vi "DIO_PWM_Encoder_I2C.vi"(0 "DIO.1:0.OUT":fxp<+,2,2> format="%.0b", 1 "DIO.1:0.DIR":fxp<+,2,2> format="%.0b", 3 "PWM.GROUP IN":T3 {"PWM.1.CNFG" format="%08b"; "PWM.0.CNFG" format="%08b"}, 4 "Encoder.GROUP IN":T4 {"ENC.STAT" format="%08b"}, 5 "I2C.GROUP IN":T1={"I2C.GO"=FALSE, "I2C.CNFG"=1, "I2C.DATO"=0, "I2C.DATI"=0, "I2C.ADDR"=0, "I2C.CNTR"=213, "I2C.CNTL"=0, "I2C.STAT"=0} {"I2C.STAT" format="%08b"; "I2C.CNTL" format="%08b"; "I2C.ADDR" format="%08b"; "I2C.CNFG" format="%08b"}, 6 "DIO0/PWM0/ENC.A/I2C.SCL Refnum":refnum<k21>, 7 "DIO.1:0.Selector":fxp<+,4,4> format="%.0b", 8 "DIO1/PWM1/ENC.B/I2C.SDA Refnum":refnum<k21>) -> (14 "IN 1:0":fxp<+,2,2> format="%02b", 17 "PWM.GROUP OUT":T3 {"PWM.1.CNFG" format="%08b"; "PWM.0.CNFG" format="%08b"}, 18 "Encoder.GROUP OUT":T4 {"ENC.STAT" format="%08b"}, 19 "I2C.GROUP OUT":T1={"I2C.GO"=FALSE, "I2C.CNFG"=1, "I2C.DATO"=0, "I2C.DATI"=0, "I2C.ADDR"=0, "I2C.CNTR"=213, "I2C.CNTL"=0, "I2C.STAT"=0} {"I2C.STAT" format="%08b"; "I2C.CNTL" format="%08b"; "I2C.ADDR" format="%08b"; "I2C.CNFG" format="%08b"})   [LabVIEW 2019]
uses:
  Utilities/PWM Configuration Group.ctl
  Utilities/Encoder Configuration Group.ctl
  Utilities/I2C Configuration Group.ctl
  Utilities/Start Boolean.ctl
  <vilib>/rvi/eio/common/nirviEmuTemplateMethod_errors.vi
  <vilib>/eio/EIONode/EIONode.xnode
panel:
  # "This VI switches between the DIO functionality and the PWM/Encoder/I2C functionality for the specified FPGA I/O channels. Each bit has a selector which contains two-bits booleans.\n- If SELECT 0 is 00, DIO enabled.\n- If SELECT 0 is 01, PWM enabled.\n- If SELECT 0 is 10, Encoder enabled.\n- If SELECT 0 is 11, I2C enabled."
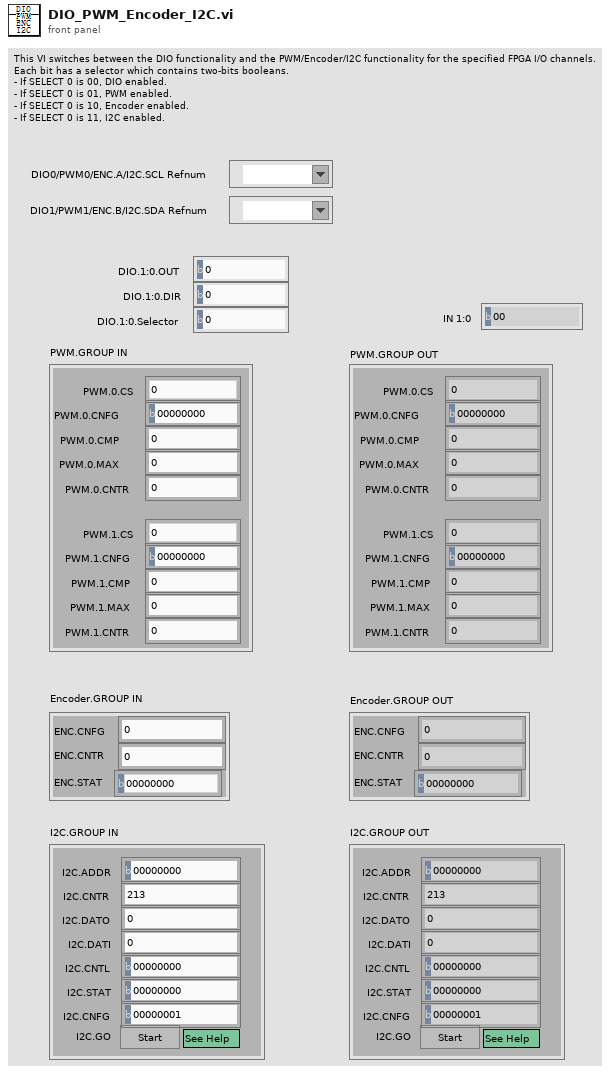
[diagram p1: front panel]
types:
  T1 = typedef "I2C Configuration Group.ctl" = cluster{"I2C.GO":T2, "I2C.CNFG":u8, "I2C.DATO":u8, "I2C.DATI":u8, "I2C.ADDR":u8, "I2C.CNTR":u8, "I2C.CNTL":u8, "I2C.STAT":u8}
  T2 = typedef "Start Boolean.ctl" = bool
  T3 = typedef "PWM Configuration Group.ctl" = cluster{"PWM.0.CS":u8, "PWM.0.CNFG":u8, "PWM.0.CMP":u16, "PWM.0.MAX":u16, "PWM.0.CNTR":u16, "PWM.1.CS":u8, "PWM.1.CNFG":u8, "PWM.1.CMP":u16, "PWM.1.MAX":u16, "PWM.1.CNTR":u16}
  T4 = typedef "Encoder Configuration Group.ctl" = cluster{"ENC.CNFG":u8, "ENC.CNTR":u32, "ENC.STAT":u8}
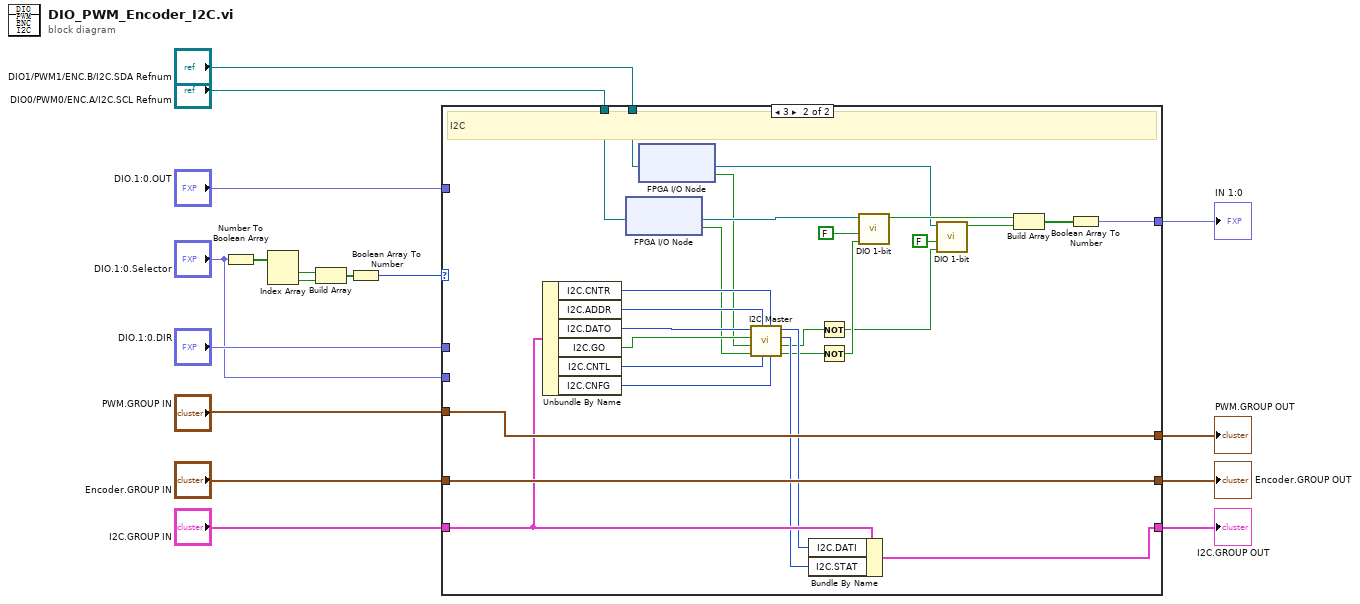
[diagram p0: block diagram]
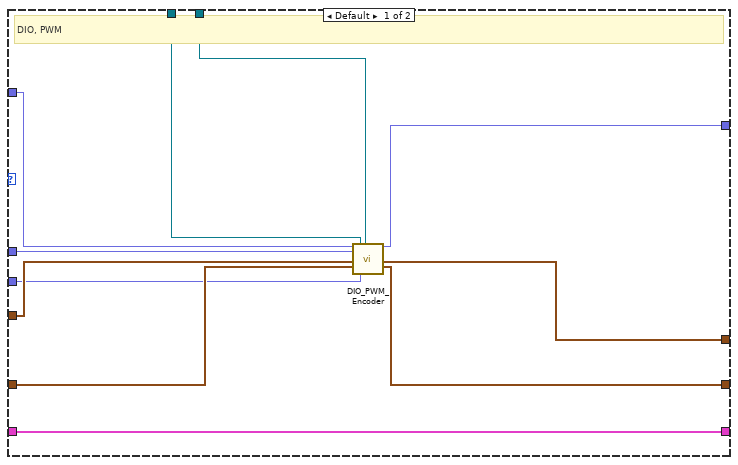
[diagram p2: hidden frame]
diagram:
  n1 = Number To Boolean Array(number="DIO.1:0.Selector") -> (Boolean array=w17:bool[])
  n2 = Index Array(array=w17) -> (element #1=w6:bool, element #2=w16:bool)  [unwired: 2 in]
  n3 = Build Array(w6, w16) -> (w15:bool[])
  n4 = Boolean Array To Number(Boolean array=w15) -> (number=w11:u8)
  n5 = case shown="3" w11 {
    tunnel: "PWM.GROUP IN" -> [w25 w55]
    tunnel: "Encoder.GROUP IN" -> [w24 w56]
    tunnel: [w22 w55] -> w12
    tunnel: [w21 w56] -> w7
    tunnel: [w23 w37] -> w10
    tunnel: "DIO0/PWM0/ENC.A/I2C.SCL Refnum" -> [w28 w36]
    tunnel: "DIO1/PWM1/ENC.B/I2C.SDA Refnum" -> [w27 w34]
    tunnel: "I2C.GROUP IN" -> [w19 w48]
    tunnel: [w19 w47] -> w4
    tunnel: "DIO.1:0.DIR" -> [w26 _]
    tunnel: "DIO.1:0.Selector" -> [w20 _]
    tunnel: "DIO.1:0.OUT" -> [w18 _]
    frame Default {
      # "DIO, PWM"
      n6 = call "DIO_PWM_Encoder.vi"("DIO.1:0.OUT"=w18, "DIO.1:0.DIR"=w26, "PWM.GROUP IN"=w25, "Encoder.GROUP IN"=w24, "DIO0/PWM0/ENC.A Refnum"=w28, "DIO.1:0.Selector"=w20, "DIO1/PWM1/ENC.B Refnum"=w27) -> ("IN 1:0"=w23:fxp<+,2,2>, "PWM.GROUP OUT"=w22:T3, "Encoder.GROUP OUT"=w21:T4)  [unwired: 10 in]
    }
    frame 3 {
      # "I2C"
      n7 = Unbundle By Name(w48) -> ("I2C.CNTR"=w54:u8, "I2C.ADDR"=w53:u8, "I2C.DATO"=w52:u8, "I2C.GO"=w51:T2, "I2C.CNTL"=w50:u8, "I2C.CNFG"=w49:u8)
      n8 = xnode "FPGA I/O Node"("FPGA I/O输入"=w36) -> ("I/O项"=w32:bool, "FPGA I/O输出"=w35:refnum<k21>)
      n9 = xnode "FPGA I/O Node"("FPGA I/O输入"=w34) -> ("I/O项"=w31:bool, "FPGA I/O输出"=w33:refnum<k21>)
      n10 = call "I2C Master.vi"("Configuration"=w49, "Counter"=w54, "Control"=w50, "Address In"=w53, "SCL_IN"=w32, "SDA_IN"=w31, "Execute?"=w51, "Data Out"=w52) -> ("SCL_OUT"=w30:bool, "SDA_OUT"=w29:bool, "Status"=w45:u8, "Data In"=w46:u8)
      n11 = Bundle By Name(cluster=w48, "I2C.DATI"=w46, "I2C.STAT"=w45) -> (w47:T1)
      n12 = Not(x=w29) -> (.not. x?=w43:bool)
      n13 = Not(x=w30) -> (.not. x?=w44:bool)
      n14 = call "DIO 1-bit.vi"("DIR"=w44, "OUT"=FALSE, "DIO Refnum"=w35) -> ("IN"=w38:bool)  [unwired: 8 in]
      n15 = call "DIO 1-bit.vi"("DIR"=w43, "OUT"=FALSE, "DIO Refnum"=w33) -> ("IN"=w39:bool)  [unwired: 8 in]
      n16 = Build Array(w38, w39) -> (w40:bool[])
      n17 = Boolean Array To Number(Boolean array=w40) -> (number=w37:fxp<+,2,2>)
    }
  }
  "IN 1:0" <- w10
  "PWM.GROUP OUT" <- w12
  "Encoder.GROUP OUT" <- w7
  "I2C.GROUP OUT" <- w4
